vi "Event handler-VidRec enable in time series.vi"(11 "Video Record-Live Imaging.NewVal":bool) -> ()   [LabVIEW 2020]
uses:
  Typedefs/Read Write Enum.ctl
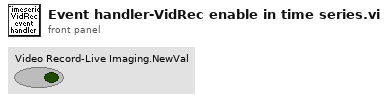
[diagram p1: front panel]
types:
  T1 = typedef "Read Write Enum.ctl" = enum16{"Read", "Write"}
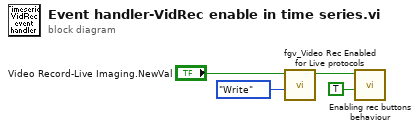
[diagram p0: block diagram]
diagram:
  n1 = call "fgv_Video Rec Enabled for Live protocols.vi"("Function"=Read_Write_Enum."Write", "Video Recording Enabled for Live protocols"="Video Record-Live Imaging.NewVal") -> ("Video Recording Enabled for Live protocols"=w3:bool)  [unwired: 9 in]
  n2 = call "Enabling rec buttons behaviour.vi"("Live img"=TRUE ("Value (Signaling)"), "New Value"=w3) -> ()  [unwired: 10 in]
